vi "ATS_MS_Set_Device_4Ch.vi"(8 "Update_Only":bool, 9 "Set_Manually (F)":bool, 10 "Setup_In":T1={"Record"={"Count"=1, "Presize"=512, "Length"=4096}, "Clock"={"ClckSource"=enum."Internal", "ClckRate"=16, "ClckEdge"=0, "Decimation"=0}, "Inputs"=[], "Trigger"={"TrigOperation"=enum."Only X", "Timeout (s)"=1.0, "Trig. Delay"=0, "Engine X"={"Source"=enum."Chan_A", "Slope"=enum."Positive", "Level"=128}, "Engine Y"={"Source"=enum."Disable", "Slope"=enum."Positive", "Level"=128}, "ExtTrigControl"={"Coupling"=enum."AC", "Range"=enum."1 V"}}} {"Inputs"."Range" items=["20mv", "40mV", "50mV", "80mV", "100mV", "200mV", "400mV", "500mV", "800mV", "1 V", "2 V", "4 V", "5 V", "8 V", "10 V", "20 V"]; "Clock"."ClckEdge" items=["Rising", "Falling"]; "Clock"."ClckRate" items=["1 kS/s", "2 kS/s", "5 kS/s", "10 kS/s", "20 kS/s", "50 kS/s", "100 kS/s", "200 kS/s", "500 kS/s", "1 MS/s", "2 MS/s", "5 MS/s", "10 MS/s", "20 MS/s", "25 MS/s", "50 MS/s", "100 MS/s", "125 MS/s", "200 MS/s", "250 MS/s", "500 MS/s", "1 GS/s"]; "Trigger"."Timeout (s)" format="%.2f"}, 11 "DeviceIn":i32) -> (0 "error out":errorcluster={"status"=TRUE, "code"=60, "source"="ATS :     ApiInvalidHandle"}, 1 "Clock_Value (s)":dbl format="%.2p", 2 "Setup_Out":T1={"Record"={"Count"=1, "Presize"=512, "Length"=4096}, "Clock"={"ClckSource"=enum."Internal", "ClckRate"=16, "ClckEdge"=0, "Decimation"=0}, "Inputs"=[], "Trigger"={"TrigOperation"=enum."Only X", "Timeout (s)"=1.0, "Trig. Delay"=0, "Engine X"={"Source"=enum."Chan_A", "Slope"=enum."Positive", "Level"=128}, "Engine Y"={"Source"=enum."Disable", "Slope"=enum."Positive", "Level"=128}, "ExtTrigControl"={"Coupling"=enum."AC", "Range"=enum."1 V"}}} {"Inputs"."Range" items=["20mv", "40mV", "50mV", "80mV", "100mV", "200mV", "400mV", "500mV", "800mV", "1 V", "2 V", "4 V", "5 V", "8 V", "10 V", "20 V"]; "Clock"."ClckEdge" items=["Rising", "Falling"]; "Clock"."ClckRate" items=["1 kS/s", "2 kS/s", "5 kS/s", "10 kS/s", "20 kS/s", "50 kS/s", "100 kS/s", "200 kS/s", "500 kS/s", "1 MS/s", "2 MS/s", "5 MS/s", "10 MS/s", "20 MS/s", "25 MS/s", "50 MS/s", "100 MS/s", "125 MS/s", "200 MS/s", "250 MS/s", "500 MS/s", "1 GS/s"]; "Trigger"."Timeout (s)" format="%.2f"}, 3 "DeviceOut":i32, 4 "TimeOut":dbl format="%.2f", 5 "#Device":i32)   [LabVIEW 2014]
doc: "_____AlazarTech, Scope_____\n\nSet ATS device with Setup_In parameters.\nIf Set_Manually is TRUE : Front panel open and the user can change setting.\nIf Set_Manually is FALSE: \n - update using input parameters.\n If UPDATE_Only is TRUE: update from previous set parameters"
uses:
  ATS_ctl/ATS_Global_4Ch.ctl
  ATS_ctl/Record.ctl
  ATS_ctl/Clock.ctl
  ATS_ctl/ClockSource.ctl
  ATS_ctl/ClockRate.ctl
  ATS_ctl/ClockEdge.ctl
  ATS_ctl/ATS_InputArray.ctl
  ATS_ctl/InputCtrl.ctl
  ATS_ctl/Coupling.ctl
  ATS_ctl/Range.ctl
  ATS_ctl/Impedance.ctl
  ATS_ctl/Bandwidth.ctl
  ATS_ctl/ATS_Trigger_4Ch.ctl
  ATS_ctl/TriggerOperation.ctl
  ATS_ctl/ATS_TriggerEngine_4Ch.ctl
  ATS_ctl/ATS_TriggerSource_4Ch.ctl
  ATS_ctl/ExtTrigger.ctl
  ATS_ctl/ExtTrigRange.ctl
  ATS_ctl/ATS_Spec_Selector.ctl
  ATS_ctl/ATS_Global_Ctrl.ctl
panel:
  out "Ch_<>":string
  out "Board":string
  out "Device":i32
  in  "String":string="Set parameters then push \"Continue ==>\""
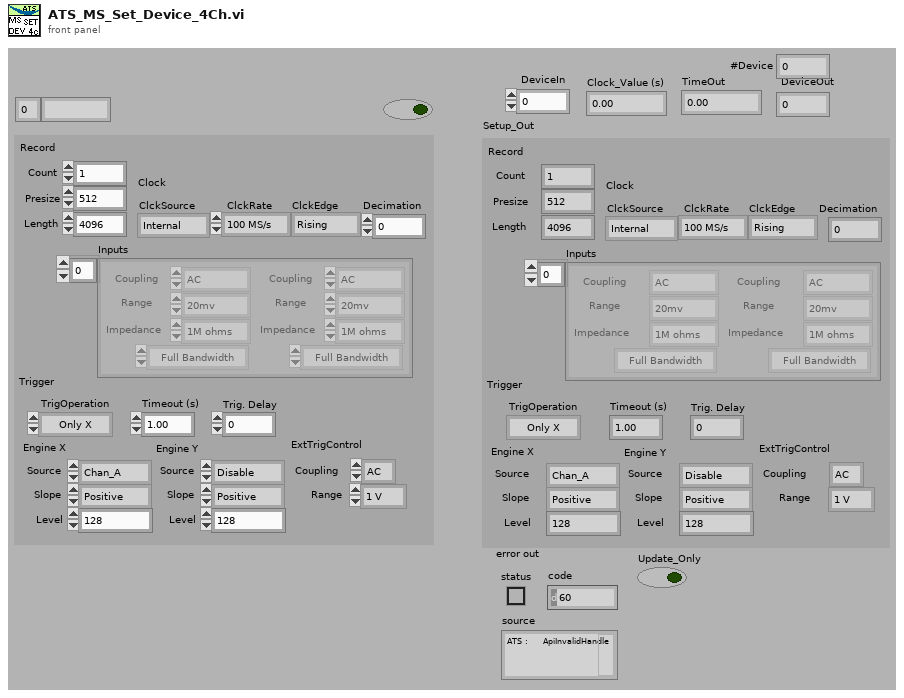
[diagram p1: front panel]
types:
  T1 = typedef "ATS_Global_4Ch.ctl" = cluster{"Record":T2, "Clock":T3, "Inputs":T7, "Trigger":T13}
  T2 = typedef "Record.ctl" = cluster{"Count":u32, "Presize":u32, "Length":u32}
  T3 = typedef "Clock.ctl" = cluster{"ClckSource":T4, "ClckRate":T5, "ClckEdge":T6, "Decimation":u32}
  T4 = typedef "ClockSource.ctl" = enum16{"Internal", "External", "Medium Ext.", "Slow Ext.", "Ext. AC", "Ext. DC", "Ext. (PLL)"}
  T5 = typedef "ClockRate.ctl" = u32
  T6 = typedef "ClockEdge.ctl" = u16
  T7 = typedef "ATS_InputArray.ctl" = T8[]
  T8 = typedef "InputCtrl.ctl" = cluster{"Coupling":T9, "Range":T10, "Impedance":T11, "Bandwidth":T12}
  T9 = typedef "Coupling.ctl" = enum16{"AC", "DC"}
  T10 = typedef "Range.ctl" = u32
  T11 = typedef "Impedance.ctl" = enum16{"1M ohms", "50 ohms"}
  T12 = typedef "Bandwidth.ctl" = enum16{"Full Bandwidth", "Reduce Bandwidth"}
  T13 = typedef "ATS_Trigger_4Ch.ctl" = cluster{"TrigOperation":T14, "Timeout (s)":dbl, "Trig. Delay":u32, "Engine X":T15, "Engine Y":T15, "ExtTrigControl":T17}
  T14 = typedef "TriggerOperation.ctl" = enum16{"Only X", "Only Y", "X or Y", "X and Y", "X xor Y", "X and not Y", "not X and Y"}
  T15 = typedef "ATS_TriggerEngine_4Ch.ctl" = cluster{"Source":T16, "Slope":enum32{"Positive", "Negative"}, "Level":u32}
  T16 = typedef "ATS_TriggerSource_4Ch.ctl" = enum32{"Chan_A", "Chan_B", "External", "Disable", "Chan_C", "Chan_D"}
  T17 = typedef "ExtTrigger.ctl" = cluster{"Coupling":T9, "Range":T18}
  T18 = typedef "ExtTrigRange.ctl" = enum16{"1 V", "5 V", "TTL"}
  T19 = typedef "ATS_Spec_Selector.ctl" = enum16{"None", "ClckSource", "ClckEdge", "ClckRate", "InputRange", "InputCoupling", "Impedance", "Bandwidth", "AsyncDMA", "Memory", "ExtTrigCoupling", "ExtTrigRange", "AUX_IO_Trig", "AUX_IO_Slope", "Trigger_Source"}
  T20 = typedef "ATS_Global_Ctrl.ctl" = enum16{"Init_Device", "Clear_ALL", "Set", "Get"}
  T21 = typedef "ATS_Global_Specs_Ctrl.ctl" = cluster{"ClckSource":cluster{"Internal":bool, "External":bool, "Medium Ext.":bool, "Slow Ext.":bool, "Ext. AC":bool, "Ext. DC":bool, "Ext. (PLL)":bool}, "ClckRate":cluster{"1 kS/s":bool, "2 kS/s":bool, "5 kS/s":bool, "10 kS/s":bool, "20 kS/s":bool, "50 kS/s":bool, "100 kS/s":bool, "200 kS/s":bool, "500 kS/s":bool, "1 MS/s":bool, "2 MS/s":bool, "5 MS/s":bool, "10 MS/s":bool, "20 MS/s":bool, "25 MS/s":bool, "50 MS/s":bool, "100 MS/s":bool, "125 MS/s":bool, "160 MS/s":bool, "180 MS/s":bool, "200 MS/s":bool, "250 MS/s":bool, "500 MS/s":bool, "1 GS/s":bool}, "ClckEdge":cluster{"Rising":bool, "Falling":bool}, "InputCoupling":cluster{"AC":bool, "DC":bool}, "InputRange":cluster{"20mV":bool, "40mV":bool, "50mV":bool, "80mV":bool, "100mV":bool, "200mV":bool, "400mV":bool, "500mV":bool, "800mV":bool, "1 V":bool, "2 V":bool, "4 V":bool, "5 V":bool, "8 V":bool, "10 V":bool, "16 V":bool, "20 V":bool, "40 V":bool, "HiFi":bool, "1.25 V":bool}, "Impedance":cluster{"1M ohms":bool, "50 ohms":bool, "300 ohms":bool}, "Bandwidth":cluster{"Full":bool, "Reduce":bool}, "RangeLim(50)":string, "AsyncDMA":cluster{"OnBoard":bool, "FPGA":bool}, "Memory":cluster{"VerifMem":bool, "HighMem":bool, "Combine":bool, "HighRecord":bool}, "ExtTrigCoupling":cluster{"AC":bool, "DC":bool}, "ExtTrigRange":cluster{"1 V":bool, "5 V":bool, "\nTTL":bool}, "AUX_IO_Trig":cluster{"Trig_Out":bool, "Trig_In":bool}, "AUX_IO_Slope":cluster{"Rising":bool, "Falling":bool}, "MaxPretrig":cluster{"MEM":u32, "FIFO":u32}, "AUX_I/O_Trig":cluster{"OUT_Trigger":bool, "OUT_PACER":bool, "OUT_BUSY":bool, "OUT_CLOCK":bool, "OUT_RESERVED":bool, "OUT_CAPTURE_ALMOST_DONE":bool, "OUT_AUXILIARY":bool, "OUT_SERIAL_DATA":bool, "IN_TRIGGER_ENABLE":bool, "IN_DIGITAL_TRIGGER":bool, "IN_GATE":bool, "IN_CAPTURE_ON_DEMAND":bool, "IN_RESET_TIMESTAMP":bool, "IN_SLOW_EXTERNAL_CLOCK":bool, "INPUT_AUXILIARY":bool, "INPUT_SERIAL_DATA":bool}, "ChannelsPerBoard":u8}
  T22 = typedef "Device_Info.ctl" = cluster{"Handle":u32, "Board":string, "CPLD":string, "MemorySize":u32, "SampleSize":u8, "ID":i32, "High_Memory":bool, "Chan/Board":u8}
  T23 = typedef "ATS_Sys_Info.ctl" = cluster{"MS_Mode":bool, "MBoard":i32, "#Board":i32}
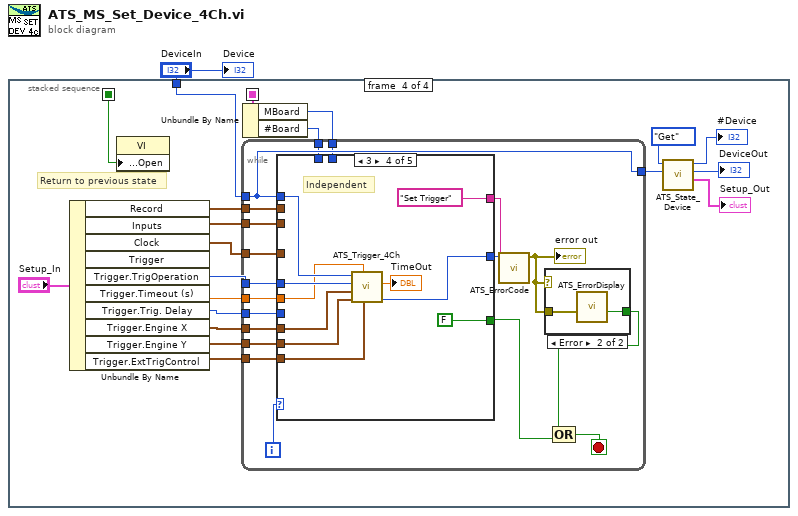
[diagram p0: block diagram]
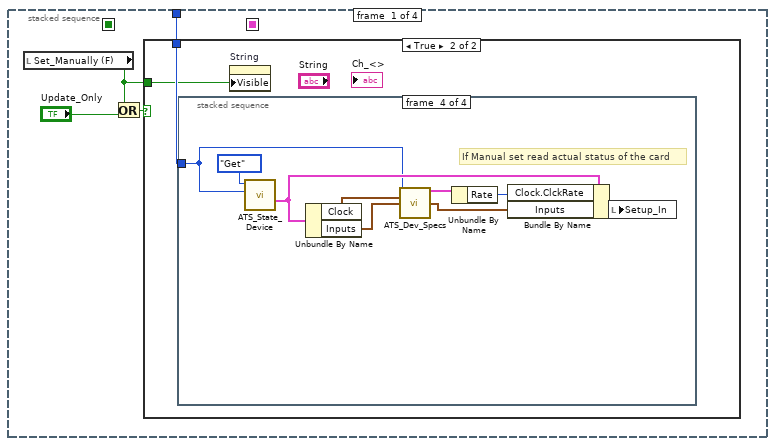
[diagram p2: hidden frame]
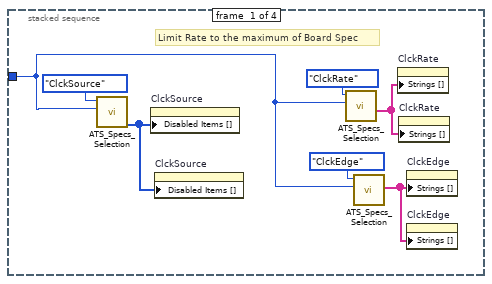
[diagram p4: hidden frame]
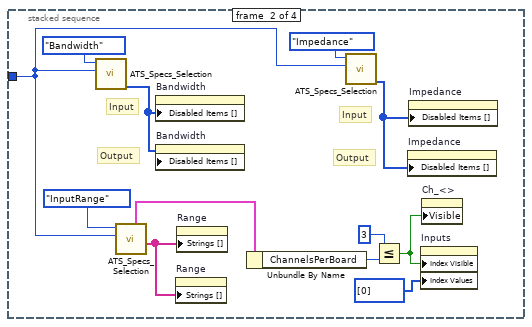
[diagram p5: hidden frame]
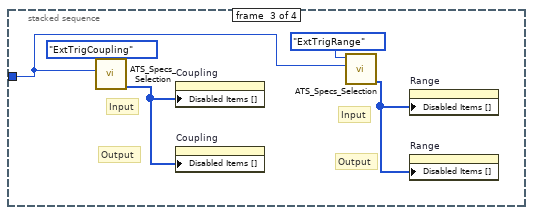
[diagram p6: hidden frame]
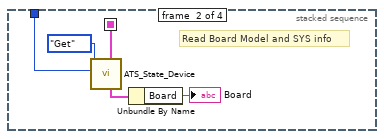
[diagram p7: hidden frame]
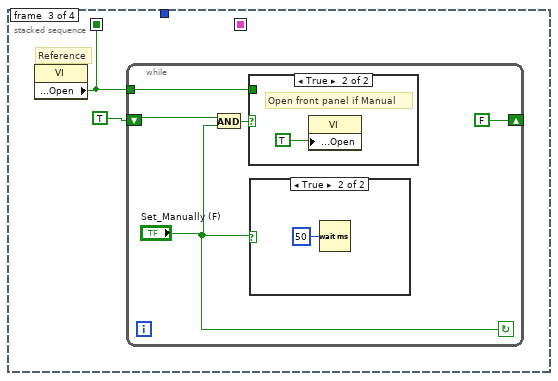
[diagram p8: hidden frame]
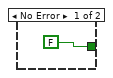
[diagram p11: hidden frame]
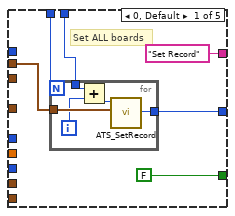
[diagram p12: hidden frame]
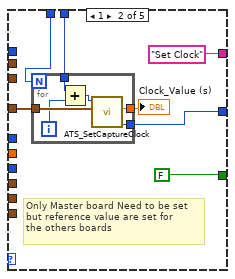
[diagram p13: hidden frame]
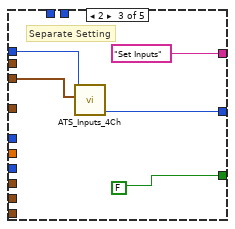
[diagram p14: hidden frame]
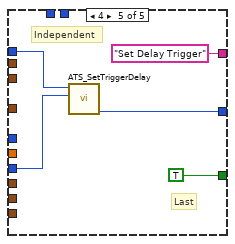
[diagram p15: hidden frame]
diagram:
  n1 = stacked-sequence {
    seq-local: [_ _ w46 _] -> [_ _ _ w64]
    seq-local: [_ w42 _ _] -> [_ _ _ w55]
    tunnel: "DeviceIn" -> [w5 w41 _ w58]
    frame #0 {
      n2 = local read "Set_Manually (F)"() -> (w2:bool)
      n3 = Or(x=w2, y="Update_Only") -> (x .or. y?=w4:bool)
      n4 = case shown="True" w4 {
        tunnel: w5 -> [_ w7]
        tunnel: w2 -> [_ w6]
        frame False {
        }
        frame True {
          n5 = stacked-sequence {
            tunnel: w7 -> [w10 w23 w29 w34]
            frame #0 {
              # "Limit Rate to the maximum of Board Spec"
              n6 = call "ATS_Specs_Selection.vi"("Device"=w10, "ATS_Spec_Selector"=ATS_Spec_Selector."ClckSource") -> ("Disabled_Item"=w9:i32[])  [unwired: 3 in, 6 out]
              n7 = property on="ClckSource" class="Enum (strict)"("Disabled Items []"=w9) -> ()  [unwired: 2 in, 2 out]
              n8 = property on="ClckSource" class="Enum (strict)"("Disabled Items []"=w9) -> ()  [unwired: 2 in, 2 out]
              n9 = call "ATS_Specs_Selection.vi"("Device"=w10, "ATS_Spec_Selector"=ATS_Spec_Selector."ClckRate") -> ("Possible_Item"=w14:string[])  [unwired: 3 in, 6 out]
              n10 = call "ATS_Specs_Selection.vi"("Device"=w10, "ATS_Spec_Selector"=ATS_Spec_Selector."ClckEdge") -> ("All_Item"=w8:string[])  [unwired: 3 in, 6 out]
              n11 = property on="ClckRate" class="Ring (strict)"("Strings []"=w14) -> ()  [unwired: 2 in, 2 out]
              n12 = property on="ClckRate" class="Ring (strict)"("Strings []"=w14) -> ()  [unwired: 2 in, 2 out]
              n13 = property on="ClckEdge" class="Ring (strict)"("Strings []"=w8) -> ()  [unwired: 2 in, 2 out]
              n14 = property on="ClckEdge" class="Ring (strict)"("Strings []"=w8) -> ()  [unwired: 2 in, 2 out]
            }
            frame #1 {
              # "Output"
              # "Input"
              # "Output"
              # "Input"
              n15 = call "ATS_Specs_Selection.vi"("Device"=w23, "ATS_Spec_Selector"=ATS_Spec_Selector."Bandwidth") -> ("Disabled_Item"=w17:i32[])  [unwired: 3 in, 6 out]
              n16 = call "ATS_Specs_Selection.vi"("Device"=w23, "ATS_Spec_Selector"=ATS_Spec_Selector."InputRange") -> ("Possible_Item"=w18:string[], "Specifications"=w19:T21)  [unwired: 3 in, 5 out]
              n17 = property on="Bandwidth" class="Enum (strict)"("Disabled Items []"=w17) -> ()  [unwired: 2 in, 2 out]
              n18 = property on="Bandwidth" class="Enum (strict)"("Disabled Items []"=w17) -> ()  [unwired: 2 in, 2 out]
              n19 = property on="Range" class="Ring (strict)"("Strings []"=w18) -> ()  [unwired: 2 in, 2 out]
              n20 = property on="Range" class="Ring (strict)"("Strings []"=w18) -> ()  [unwired: 2 in, 2 out]
              n21 = Unbundle By Name(w19) -> ("ChannelsPerBoard"=w21:u8)
              n22 = call "ATS_Specs_Selection.vi"("Device"=w23, "ATS_Spec_Selector"=ATS_Spec_Selector."Impedance") -> ("Disabled_Item"=w16:i32[])  [unwired: 3 in, 6 out]
              n23 = Less Or Equal?(x=u8 3, y=w21) -> (x <= y?=w15:bool)
              n24 = property on="Impedance" class="Enum (strict)"("Disabled Items []"=w16) -> ()  [unwired: 2 in, 2 out]
              n25 = property on="Impedance" class="Enum (strict)"("Disabled Items []"=w16) -> ()  [unwired: 2 in, 2 out]
              n26 = property on="Inputs" class="Arr (strict)"("Index Visible"=w15, "Index Values"=u32[] [0]) -> ()  [unwired: 2 in, 2 out]
              n27 = property on="Ch_<>" class="Str"("Visible"=w15) -> ()  [unwired: 2 in, 2 out]
            }
            frame #2 {
              # "Output"
              # "Input"
              # "Output"
              # "Input"
              n28 = call "ATS_Specs_Selection.vi"("Device"=w29, "ATS_Spec_Selector"=ATS_Spec_Selector."ExtTrigCoupling") -> ("Disabled_Item"=w28:i32[])  [unwired: 3 in, 6 out]
              n29 = property on="Coupling" class="Enum (strict)"("Disabled Items []"=w28) -> ()  [unwired: 2 in, 2 out]
              n30 = property on="Coupling" class="Enum (strict)"("Disabled Items []"=w28) -> ()  [unwired: 2 in, 2 out]
              n31 = call "ATS_Specs_Selection.vi"("Device"=w29, "ATS_Spec_Selector"=ATS_Spec_Selector."ExtTrigRange") -> ("Disabled_Item"=w27:i32[])  [unwired: 3 in, 6 out]
              n32 = property on="Range" class="Enum (strict)"("Disabled Items []"=w27) -> ()  [unwired: 2 in, 2 out]
              n33 = property on="Range" class="Enum (strict)"("Disabled Items []"=w27) -> ()  [unwired: 2 in, 2 out]
            }
            frame #3 {
              # "If Manual set read actual status of the card"
              n34 = call "ATS_State_Device.vi"("DeviceIn"=w34, "ATS_GBL_Ctrl"=ATS_Global_Ctrl."Get") -> ("SetupOut"=w39:T1)  [unwired: 4 in, 5 out]
              n35 = Unbundle By Name(w39) -> ("Clock"=w36:T3, "Inputs"=w33:T7)
              n36 = call "ATS_Dev_Specs.vi"("Device"=w34, "Clock"=w36, "Input_Chan"=w33) -> ("Rate_Out"=w35:cluster{"Text":string, "Rate":i32}, "Output_Chan"=w32:T8[])  [unwired: 8 in, 3 out]
              n37 = Unbundle By Name(w35) -> ("Rate"=w38:i32)
              n38 = Bundle By Name(cluster=w39, "Clock.ClckRate"=w38, "Inputs"=w32) -> (w37:T1)
              n39 = local write "Setup_In"(w37) -> ()
            }
          }
          n40 = property on="String" class="Str"("Visible"=w6) -> ()  [unwired: 2 in, 2 out]
        }
      }
    }
    frame #1 {
      # "Read Board Model and SYS info"
      n41 = call "ATS_State_Device.vi"("DeviceIn"=w41, "ATS_GBL_Ctrl"=ATS_Global_Ctrl."Get") -> ("DevInfo_Out"=w45:T22, "Sys_Out"=w42:T23)  [unwired: 4 in, 4 out]
      n42 = Unbundle By Name(w45) -> ("Board"=→"Board":string)
    }
    frame #2 {
      # "Reference"
      n43 = property class="VI"() -> ("Front Panel Window:Open"=w46:bool)  [unwired: 2 in, 2 out]
      n44 = while {
        shift-right: [FALSE ("Front Panel Window:Open")] -> _
        shift-left: TRUE ("Front Panel Window:Open") -> [w51]
        tunnel: w46 -> [w50]
        stop <- "Set_Manually (F)" continue-if-true
        n45 = And(x=w51, y="Set_Manually (F)") -> (x .and. y?=w49:bool)
        n46 = case shown="True" w49 {
          tunnel: w50 -> [_ _]
          frame False {
          }
          frame True {
            # "Open front panel if Manual"
            n47 = property class="VI"("Front Panel Window:Open"=TRUE) -> ()  [unwired: 2 in, 2 out]
          }
        }
        n48 = case shown="True" "Set_Manually (F)" {
          frame False {
            # "No Stop"
          }
          frame True {
            n49 = Wait (ms)(milliseconds to wait=u32 50) -> ()  [unwired: 1 out]
          }
        }
      }
    }
    frame #3 {
      # "Return to previous state"
      n50 = Unbundle By Name("Setup_In") -> ("Record"=w73:T2, "Inputs"=w71:T7, "Clock"=w72:T3, "Trigger.TrigOperation"=w67:T14, "Trigger.Timeout (s)"=w66:dbl, "Trigger.Trig. Delay"=w65:u32, "Trigger.Engine X"=w68:T15, "Trigger.Engine Y"=w69:T15, "Trigger.ExtTrigControl"=w70:T17)  [unwired: 1 out]
      n51 = property class="VI"("Front Panel Window:Open"=w64) -> ()  [unwired: 2 in, 2 out]
      n52 = Unbundle By Name(w55) -> ("MBoard"=w57:i32, "#Board"=w56:i32)
      n53 = while {
        tunnel: w58 -> [w81]
        tunnel: w73 -> [w90]
        tunnel: w72 -> [w89]
        tunnel: w71 -> [w88]
        tunnel: w70 -> [w87]
        tunnel: w69 -> [w86]
        tunnel: w68 -> [w85]
        tunnel: w67 -> [w84]
        tunnel: w66 -> [w83]
        tunnel: w65 -> [w82]
        tunnel: [w81] -> w63
        tunnel: w57 -> [w76]
        tunnel: w56 -> [w75]
        i -> [w77]
        stop <- w80 stop-if-true
        n54 = case shown="3" w77 {
          tunnel: [w102 w114 w124 w133 w140] -> w93
          tunnel: w81 -> [_ _ w125 w134 w138]
          tunnel: [FALSE ("value") FALSE ("value") FALSE ("value") FALSE ("value") TRUE ("value")] -> w79
          tunnel: w90 -> [w100 _ _ _ _]
          tunnel: w89 -> [_ w112 _ _ _]
          tunnel: w88 -> [_ _ w122 _ _]
          tunnel: w87 -> [_ _ _ w132 _]
          tunnel: w86 -> [_ _ _ w131 _]
          tunnel: w85 -> [_ _ _ w130 _]
          tunnel: w84 -> [_ _ _ w129 _]
          tunnel: w83 -> [_ _ _ w128 _]
          tunnel: w82 -> [_ _ _ _ w137]
          tunnel: ["Set Record" "Set Clock" "Set Inputs" "Set Trigger" "Set Delay Trigger"] -> w78
          tunnel: w76 -> [w98 w109 _ _ _]
          tunnel: w75 -> [w97 w108 _ _ _]
          frame 0, Default {
            # "Set ALL boards"
            n55 = for {
              N: w97 -> [_]
              tunnel: [w107] -> w102
              tunnel: w100 -> [w106]
              tunnel: w98 -> [w103]
              i -> [w104]
              n56 = Add(x=w103, y=w104) -> (x+y=w105:i32)
              n57 = call "ATS_SetRecord.vi"("RecordIn"=w106, "DeviceIn"=w105) -> ("Return Code"=w107:u32)  [unwired: 7 in, 2 out]
            }
          }
          frame 1 {
            # "Only Master board Need to be set\nbut reference value are set for\nthe others boards"
            n58 = for {
              N: w108 -> [_]
              tunnel: [w120] -> w114
              tunnel: w112 -> [w119]
              tunnel: [w118] -> w111
              tunnel: w109 -> [w115]
              i -> [w117]
              n59 = Add(x=w115, y=w117) -> (x+y=w116:i32)
              n60 = call "ATS_SetCaptureClock.vi"("Clock"=w119, "DeviceIn"=w116) -> ("Return Code"=w120:u32, "Clock_Value (s)"=w118:dbl)  [unwired: 7 in, 1 out]
            }
            "Clock_Value (s)" <- w111
          }
          frame 2 {
            # "Separate Setting"
            n61 = call "ATS_Inputs_4Ch.vi"("Channels_Input"=w122, "DeviceIn"=w125) -> ("Return Code"=w124:u32)  [unwired: 5 in, 4 out]
          }
          frame 3 {
            # "Independent"
            n62 = call "ATS_Trigger_4Ch.vi"("ExtTrigControl"=w132, "Timeout (-1, Auto)"=w128, "Engine Y"=w131, "Engine X"=w130, "TrigOperation"=w129, "DeviceIn"=w134) -> ("Return Code"=w133:u32, "Timeout"=→"TimeOut":dbl)  [unwired: 3 in, 1 out]
          }
          frame 4 {
            # "Last"
            # "Independent"
            n63 = call "ATS_SetTriggerDelay.vi"("Delay"=w137, "DeviceIn"=w138) -> ("Return Code"=w140:u32)  [unwired: 8 in, 1 out]
          }
        }
        n64 = call "ATS_ErrorCode.vi"("Message"=w78, "ErrorCode"=w93) -> ("error out"=w91:errorcluster)  [unwired: 5 in]
        "error out" <- w91
        n65 = case shown="Error" w91 {
          tunnel: [FALSE ("End 2") w96] -> w92
          tunnel: w91 -> [_ w95]
          frame No Error {
          }
          frame Error {
            n66 = call "ATS_ErrorDisplay.vi"("error IN"=w95) -> ("End Out"=w96:bool)  [unwired: 6 in]
          }
        }
        n67 = Compound Arithmetic op=OR(w92, w79) -> (w80:bool)
      }
      n68 = call "ATS_State_Device.vi"("DeviceIn"=w63, "ATS_GBL_Ctrl"=ATS_Global_Ctrl."Get") -> ("SetupOut"=→"Setup_Out":T1, "DeviceOut"=→"DeviceOut":i32, "#Device"=→"#Device":i32)  [unwired: 4 in, 3 out]
    }
  }
  "Device" <- "DeviceIn"
